vi "GetComicNameAndFolder.vi"(9 "Local Path":path=path "C:/data/comics/comics", 11 "URL":string) -> (1 "OwningFolder":path, 3 "FileName":string)   [LabVIEW 2022 SP3]
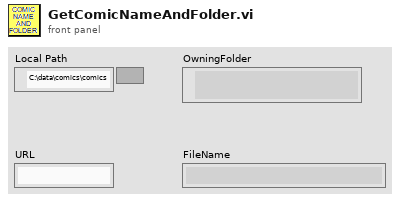
[diagram p1: front panel]
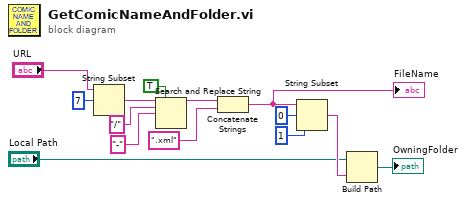
[diagram p0: block diagram]
diagram:
  n1 = String Subset(string="URL", offset (0)=7) -> (substring=w3:string)  [unwired: 1 in]
  n2 = Search and Replace String(replace all?=TRUE ("replace all? (F)"), input string=w3, search string="/", replace string="-" ("replace string (\"\")")) -> (result string=w7:string)  [unwired: 4 in, 3 out]
  n3 = Concatenate Strings(w7, ".xml" ("string")) -> (w9:string)
  "FileName" <- w9
  n4 = String Subset(string=w9, offset (0)=0, length (rest)=1 ("length (rest)")) -> (substring=w13:string)
  n5 = Build Path(base path="Local Path", name or relative path=w13) -> (appended path=→"OwningFolder":path)
